vi "Renishaw-XL80_GetIsConnect.vi"(8 "error in (no error)":errorcluster, 11 "Renishaw-XL80 in":refnum<class "Renishaw-XL80.lvclass">) -> (0 "error out":errorcluster, 2 "IsConnected":bool, 3 "Renishaw-XL80 out":refnum<class "Renishaw-XL80.lvclass">)   [LabVIEW 2024, in "Renishaw-XL80.lvclass"]
doc: "This read only property returns VARIANT_TRUE if the client has connected to a DX10 and returns VARIANT_FALSE otherwise.\n\nDefinition\nHRESULT\nget_IsConnected(\n [out, retval] VARIANT_BOOL* pVal\n);\n\nParameters\npVal\nA variable that will be set to VARIANT_TRUE or VARIANT_FALSE. \nComments\nIf this property sets pVal to VARIANT_FALSE then this indicates that either the client has not called Connect, or that the client called Connect and the method failed to find an available DX10. The property will also set pVal to VARIANT_FALSE if the client has previously called Disconnect.\n\nThe property will normally return an HRESULT of S_OK. However, it will return E_POINTER if the client supplies a null pointer for pVal."
uses:
  Renishaw-XL80.lvclass
  Renishaw-XL80.lvclass/Renishaw-XL80.ctl
  D:/A.C.M/Example CSharp_64/bin/Debug/Interop.DX10SDKADAPTORLib.dll
  Example CSharp_64/bin/Debug/Interop.DX10SDKADAPTORLib.dll
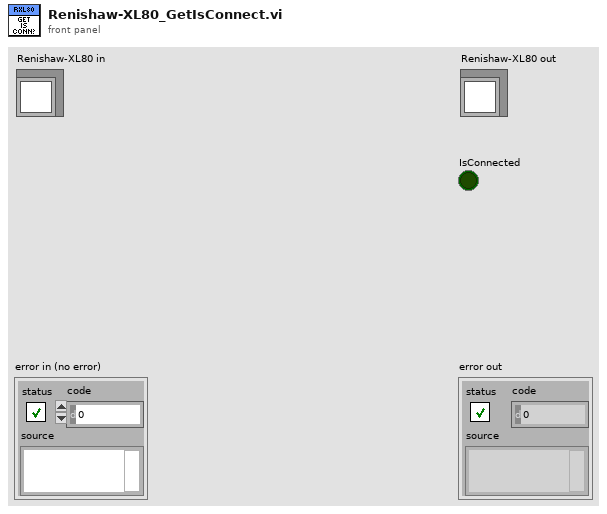
[diagram p1: front panel]
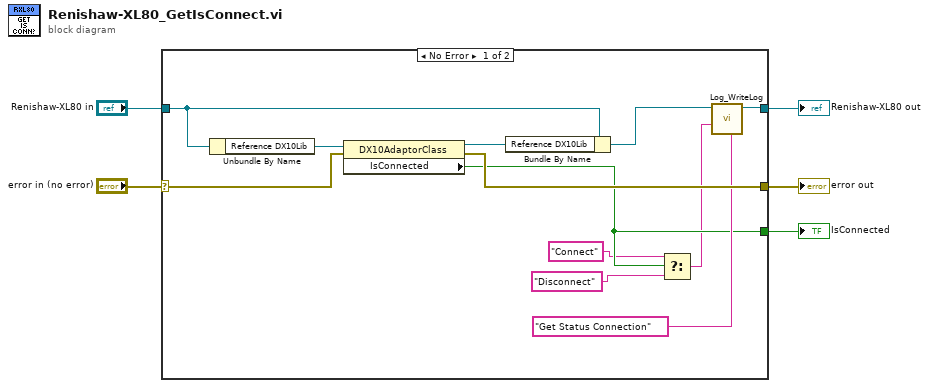
[diagram p0: block diagram]
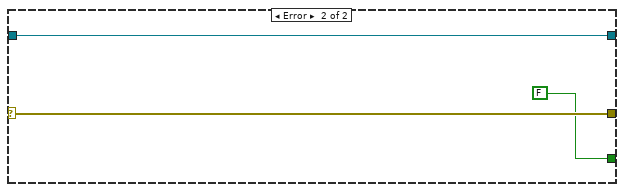
[diagram p2: hidden frame]
diagram:
  n1 = case shown="No Error" "error in (no error)" {
    selector: "error in (no error)" -> [w14 w20]
    tunnel: [w13 w20] -> w4
    tunnel: [w12 w19] -> w2
    tunnel: "Renishaw-XL80 in" -> [w15 w19]
    tunnel: [w9 FALSE ("IsConnected")] -> w1
    frame No Error {
      n2 = Unbundle By Name(w15) -> ("Reference DX10Lib"=w17:refnum<k24>)
      n3 = property class="DX10AdaptorClass"(reference=w17, error in=w14) -> (reference out=w16:refnum<k24>, error out=w13:errorcluster, "IsConnected"=w9:bool)
      n4 = Bundle By Name(cluster=w15, "Reference DX10Lib"=w16) -> (w11:refnum<class "Renishaw-XL80.lvclass">)
      n5 = Select(t="Connect" ("Additional text"), s=w9, f="Disconnect" ("Additional text")) -> (s? t:f=w6:string)
      n6 = call-dynamic "Log_WriteLog.vi"("Additional text"="Get Status Connection", "Response"=w6, "Log in"=w11) -> ("Log out"=w12:refnum<class "Renishaw-XL80.lvclass">)  [unwired: 7 in, 1 out]
    }
    frame Error {
    }
  }
  "error out" <- w4
  "Renishaw-XL80 out" <- w2
  "IsConnected" <- w1
